vi "Exe Arduino Servo Motor-Pin --LINX--.vi"(1 "Motor Name":enum8{"B", "S", "E", "C"}(ring)=enum."E") -> (0 "Pin":u8)   [LabVIEW 2015]
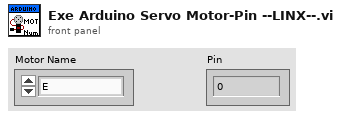
[diagram p1: front panel]
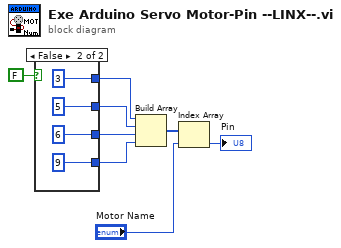
[diagram p0: block diagram]
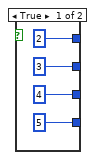
[diagram p2: hidden frame]
diagram:
  n1 = case shown="False" FALSE {
    tunnel: [u8 2 ("Pin 2") u8 3 ("Pin 2")] -> w8
    tunnel: [u8 3 ("Pin 2") u8 5 ("Pin 2")] -> w7
    tunnel: [u8 4 ("Pin 2") u8 6 ("Pin 2")] -> w6
    tunnel: [u8 5 ("Pin 2") u8 9 ("Pin 2")] -> w5
    frame True {
    }
    frame False {
    }
  }
  n2 = Build Array(w8, w7, w6, w5) -> (w4:u8[])
  n3 = Index Array(array=w4, index="Motor Name") -> (element=→"Pin":u8)
